vi "arrayexample2.vi"() -> ()   [LabVIEW 2015]
panel:
  in  "stop":bool
  out "Array 6":dbl[][](array[numeric])
  in  "Long Column":i32
  in  "Index Column":i32
  in  "Long Fila":i32
  in  "Index Fila":i32
  out "Array 5":dbl[](array[numeric])
  in  "Fila":i16
  out "Elemento":dbl
  in  "Columna":i32
  in  "Fila":i32
  out "Array 4":dbl[][](array[numeric])
  in  "Array 3":dbl[](array[numeric])
  in  "Array 2":dbl[](array[numeric])
  in  "Array":dbl[](array[numeric])
  # "IndexFila"
  # "IndexColumn"
  # "Seleecione una fila de la matriz"
  # "Seleccione un elemento de la matriz"
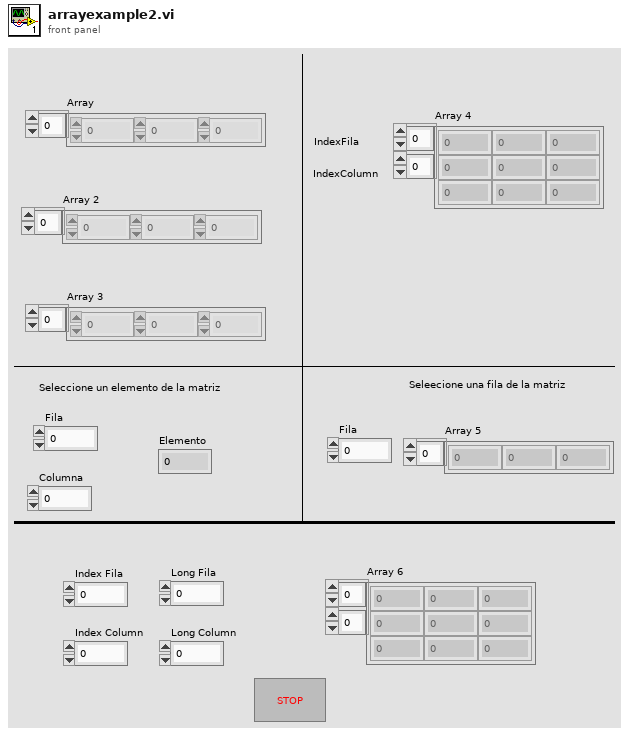
[diagram p1: front panel]
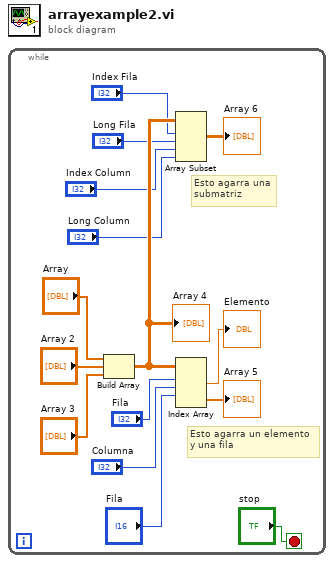
[diagram p0: block diagram]
diagram:
  n1 = while {
    stop <- "stop" stop-if-true
    # "Esto agarra un elemento\ny una fila"
    # "Esto agarra una\nsubmatriz"
    n2 = Build Array("Array", "Array 2", "Array 3") -> (w6:dbl[][])
    "Array 4" <- w6
    n3 = Array Subset(array=w6, index (row)="Index Fila", length (row)="Long Fila", index (col)="Index Column", length (col)="Long Column") -> (→"Array 6":dbl[][])
    n4 = Index Array(array=w6, index (row) #1="Fila", index (col) #1="Columna", index (row) #2="Fila") -> (element #1=→"Elemento":dbl, element #2=→"Array 5":dbl[])  [unwired: 1 in]
  }
